vi "File.Build File Name with Timestamp.vi"(7 "Time":timestamp, 10 "Sufix":string, 11 "File Name":string) -> (2 "Time Stamp Out":string, 3 "File Name Out":string)   [LabVIEW 2024]
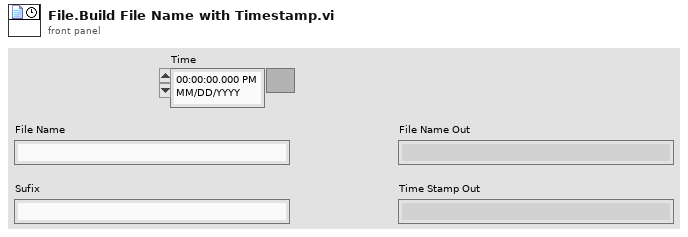
[diagram p1: front panel]
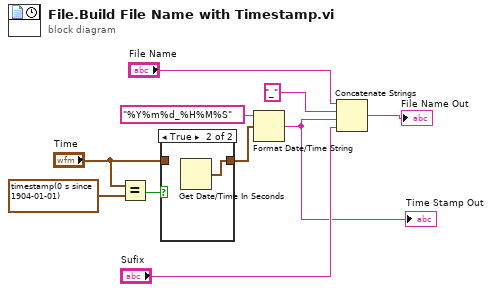
[diagram p0: block diagram]
diagram:
  n1 = Equal?(x="Time", y=timestamp(0 s since 1904-01-01) ("Time")) -> (x = y?=w3:bool)
  n2 = case shown="True" w3 {
    tunnel: "Time" -> [w11 _]
    tunnel: [w11 w12] -> w1
    frame False {
    }
    frame True {
      n3 = Get Date/Time In Seconds() -> (seconds since 1Jan1904=w12:timestamp)
    }
  }
  n4 = Format Date/Time String(time format string (%c)="%Y%m%d_%H%M%S", seconds (now)=w1) -> (date/time string=w7:string)  [unwired: 1 in]
  "Time Stamp Out" <- w7
  n5 = Concatenate Strings("File Name", "_" ("time format string (%c)"), w7, "Sufix") -> (→"File Name Out":string)
